vi "Launcher.vi"() -> ()   [LabVIEW 2016, in "Echo Broadcast Test Without Server Manager.lvlib"]
uses:
  Echo Broadcast Test Without Server Manager.lvlib
  WebSocket Actor/WebSocket Server/WebSocket Server.lvclass
  C:/Program Files (x86)/National Instruments/LabVIEW 2016/vi.lib/ActorFramework/Actor/Actor.lvclass
  WS Test Server/WS Test Server.lvclass
  WS Test Server Messages/Server Connection Handler Msg/Server Connection Handler Msg.lvclass
  C:/Projects/Shared Libraries/WebSocket Actor/WebSocket Actor/Abstract Messages/WebSocket Connection Handler Msg/WebSocket Connection Handler Msg.lvclass
  WebSocket Actor/WebSocket Server/typedefs/Listener Settings.ctl
  WebSocket Actor/WebSocket Server/WebSocket Server.lvclass/WebSocket Server.ctl
  WS Test Client/WS Test Client.lvclass
  WebSocket Actor/WebSocket Client/WebSocket Client.lvclass
  C:/Projects/Shared Libraries/WebSocket Actor/WebSocket Actor/WebSocket Connection/WebSocket Connection.lvclass
  WS Test Client Messages/Client Connection Handler Msg/Client Connection Handler Msg.lvclass
  WebSocket Actor/WebSocket Client/WebSocket Client.lvclass/WebSocket Client.ctl
  WebSocket Actor/WebSocket Connection/WebSocket Connection.lvclass/WebSocket Connection.ctl
  WebSocket Actor/WebSocket Client/properties/Write WS URI.vi
  WebSocket Actor/WebSocket Client/properties/Write Timeout (60000 ms).vi
  WebSocket Actor/WebSocket Connection/properties/Write WebSocket Data Handler.vi
  WebSocket Actor/WebSocket Server/properties/Write Listener Settings.vi
  WebSocket Actor/WebSocket Server/properties/Write Handshake timeout (5000 ms).vi
  <vilib>/ActorFramework/Actor/Actor.lvclass
  WebSocket Actor/WebSocket Server Messages/Add Service Msg/Add Service Msg.lvclass
panel:
  in  "Number of Clients":i32=3
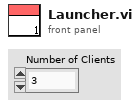
[diagram p1: front panel]
types:
  T1 = typedef "WebSocket Actors.lvlib/WebSocket Server.lvclass/Listener Settings.ctl" = cluster{"resolve remote address (T)":bool, "timeout ms (-1)":i32, "net address":u32, "port":u16}
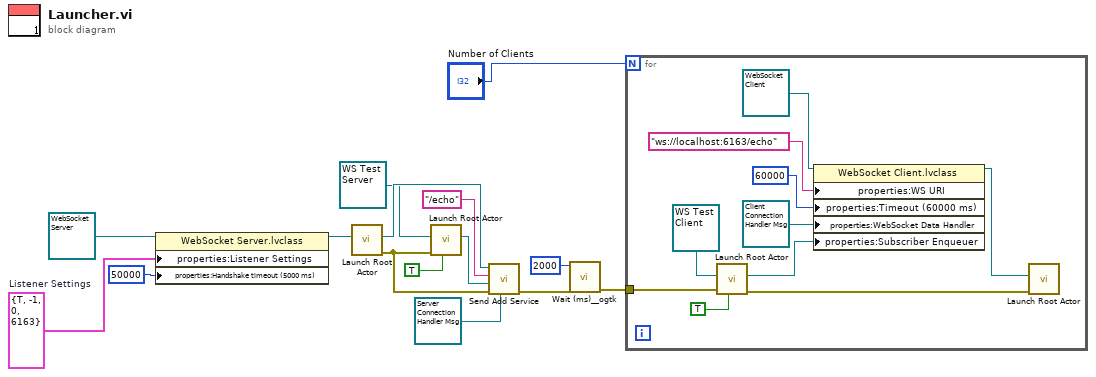
[diagram p0: block diagram]
diagram:
  w6 = T1 {"resolve remote address (T)"=TRUE, "timeout ms (-1)"=-1, "net address"=0, "port"=6163}  # Listener Settings
  n1 = property class="WebSocket Server.lvclass"(reference=refnum<class "WebSocket Server.lvclass"> refnum ("WebSocket Actors.lvlib:WebSocket Server.lvclass"), "properties:Listener Settings"=w6, "properties:Handshake timeout (5000 ms)"=50000 ("Handshake timeout (5000 ms)")) -> (reference out=w7:refnum<class "WebSocket Server.lvclass">)  [unwired: 1 in, 1 out]
  n2 = call <vilib>:"Launch Root Actor.vi"("Actor"=w7) -> ("error out"=w11:errorcluster, "Actor's Enqueuer"=w13:refnum<class "Message Enqueuer.lvclass">)  [unwired: 9 in]
  n3 = call <vilib>:"Launch Root Actor.vi"("Open Actor Core front panel? (F)"=TRUE, "error in (no error)"=w11, "Actor"=refnum<class "WS Test Server.lvclass"> refnum ("WS Full LabVIEW Test.lvlib:WS Test Server.lvclass")) -> ("Actor's Enqueuer"=w10:refnum<class "Message Enqueuer.lvclass">)  [unwired: 7 in, 1 out]
  n4 = call "Send Add Service.vi"("WebSocket Data Handler"=refnum<class "Server Connection Handler Msg.lvclass"> refnum ("WS Full LabVIEW Test.lvlib:Server Connection Handler Msg.lvclass"), "error in (no error)"=w11, "Subscriber Enqueuer"=w10, "Service Name"="/echo", "Message Enqueuer in"=w13) -> ("error out"=w2:errorcluster)  [unwired: 5 in, 1 out]
  n5 = call <userlib>:"Wait (ms)__ogtk.vi"("error in (no error)"=w2, "milliseconds to wait"=u32 2000) -> ("error out"=w1:errorcluster)  [unwired: 8 in, 1 out]
  n6 = for {
    N: "Number of Clients" -> [_]
    tunnel: w1 -> [w16]
    n7 = call <vilib>:"Launch Root Actor.vi"("Open Actor Core front panel? (F)"=TRUE, "error in (no error)"=w16, "Actor"=refnum<class "WS Test Client.lvclass"> refnum ("WS Full LabVIEW Test.lvlib:WS Test Client.lvclass")) -> ("error out"=w17:errorcluster, "Actor's Enqueuer"=w18:refnum<class "Message Enqueuer.lvclass">)  [unwired: 7 in]
    n8 = property class="WebSocket Client.lvclass"(reference=refnum<class "WebSocket Client.lvclass"> refnum ("WebSocket Actors.lvlib:WebSocket Client.lvclass"), "properties:WS URI"="ws://localhost:6163/echo" ("Address"), "properties:Timeout (60000 ms)"=60000 ("Timeout (60000 ms)"), "properties:WebSocket Data Handler"=refnum<class "Client Connection Handler Msg.lvclass"> refnum ("WS Full LabVIEW Test.lvlib:Client Connection Handler Msg.lvclass"), "properties:Subscriber Enqueuer"=w18) -> (reference out=w21:refnum<class "WebSocket Client.lvclass">)  [unwired: 1 in, 1 out]
    n9 = call <vilib>:"Launch Root Actor.vi"("error in (no error)"=w17, "Actor"=w21) -> ()  [unwired: 8 in, 2 out]
  }
